vi "New Command Status.vi"(8 "error in (no error)":errorcluster, 10 "Command Status":T1, 11 "Command Processor in":refnum<class "Command Processor.lvclass">) -> (0 "error out":errorcluster, 3 "Command Processor out":refnum<class "Command Processor.lvclass">)   [LabVIEW 2013, in "Command Processor.lvlib" / "Command Processor.lvclass"]
uses:
  Command Processor.lvclass
  Command/Command Status.ctl
  Command/State Status.ctl
  Command/Command.lvclass
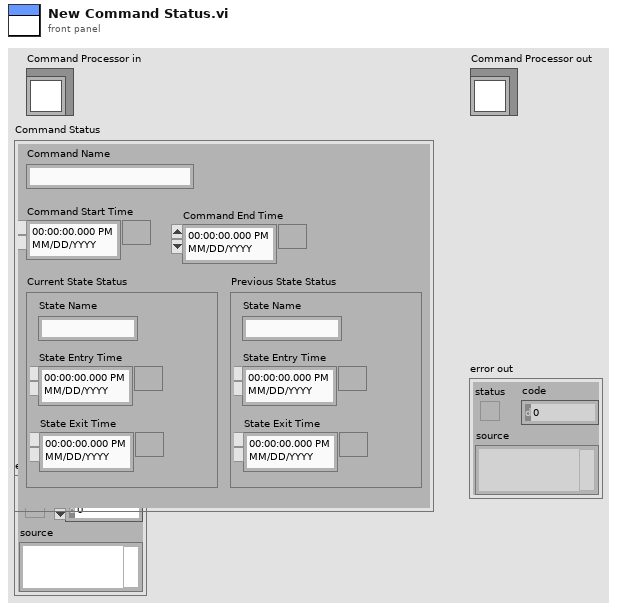
[diagram p1: front panel]
types:
  T1 = typedef "Command Processor.lvlib/Command.lvlib/Command.lvclass/Command Status.ctl" = cluster{"Command Name":string, "Current State Status":T2, "Command Start Time":timestamp, "Command End Time":timestamp, "Previous State Status":T2}
  T2 = typedef "Command Processor.lvlib/Command.lvlib/Command.lvclass/State Status.ctl" = cluster{"State Name":string, "State Entry Time":timestamp, "State Exit Time":timestamp}
  T3 = typedef "Command Processor.lvlib/Command Processor.lvclass/Command Processor Status.ctl" = cluster{"State Entry time":timestamp, "State Status":T4, "Command Processor Current State":string, "Command Status":T1}
  T4 = typedef "Current Previous State Status.ctl" = cluster{"Current State Status":T5, "Previous State Status":T5}
  T5 = typedef "State Status.ctl" = cluster{"State Name":string, "State Entry Time":timestamp, "State Exit Time":timestamp}
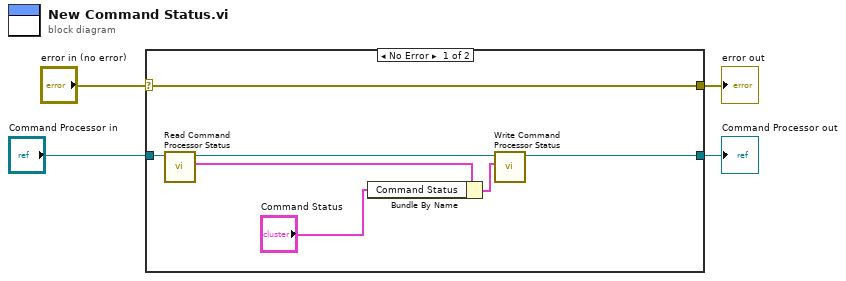
[diagram p0: block diagram]
diagram:
  n1 = case shown="No Error" "error in (no error)" {
    selector: "error in (no error)" -> [w11 w13]
    tunnel: [w11 w13] -> w3
    tunnel: [w8 w12] -> w1
    tunnel: "Command Processor in" -> [w9 w12]
    frame No Error {
      n2 = call-dynamic "Read Command Processor Status.vi"("Command Processor in"=w9) -> ("Command Processor Status"=w7:T3, "Command Processor out"=w10:refnum<class "Command Processor.lvclass">)  [unwired: 8 in, 1 out]
      n3 = Bundle By Name(cluster=w7, "Command Status"="Command Status") -> (w6:T3)
      n4 = call-dynamic "Write Command Processor Status.vi"("Command Processor Status"=w6, "Command Processor in"=w10) -> ("Command Processor out"=w8:refnum<class "Command Processor.lvclass">)  [unwired: 8 in, 1 out]
    }
    frame Error {
    }
  }
  "error out" <- w3
  "Command Processor out" <- w1
